vi "File Pwd.vi"() -> (0 "String":string="Fermion Instruments (Shanghai), Co. Ltd.")   [LabVIEW 2016, in "UserPwd DB.lvlib" / "UserPwd DB.lvclass"]
uses:
  <userlib>/Common Components/UserPwd DB/UserPwd DB/UserPwd DB.lvclass
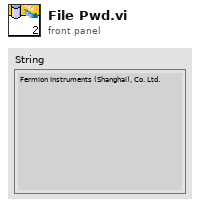
[diagram p1: front panel]
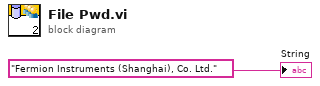
[diagram p0: block diagram]
diagram:
  "String" <- "Fermion Instruments (Shanghai), Co. Ltd."
